vi "FindPlanehs.vi"() -> ()   [LabVIEW 2022 SP3]
uses:
  <vilib>/Utility/file.llb/Write To Spreadsheet File (DBL).vi
  <vilib>/Platform/NI_3dgraph.lvlib
panel:
  in  "Save?":bool
  out "case number":i32[](graph)
  out "outer index":dbl[](array[numeric]) format="%.2f"
  in  "3D Surface":refnum<k7>(container)
  in  "Z Span (+- value range)":cluster{"x":dbl, "span":dbl, "z":dbl}={"x"=4.0, "span"=4.0, "z"=4.0} {"x" format="%.2f"; "z" format="%.2f"; "span" format="%.2f"}
  in  "Points in span":i32=10
  in  "Variables":T1={"sound spd (cm/s)"=150000, "time step (s)"=1e-08} {"time step (s)" format="%.2e"}
  in  "strip":T2={"Radius cm"=9.0, "h (cm)"=2.0, "a (cm)"=4.0} {"Radius cm" format="%.2f"; "a (cm)" format="%.2f"; "h (cm)" format="%.2f"}
  in  "P":cluster{"x cm":dbl, "y cm":dbl, "z cm":dbl}={"x cm"=0.20000000000000018, "y cm"=-4.0, "z cm"=1.4} {"x cm" format="%.2f"; "z cm" format="%.2f"; "y cm" format="%.2f"}
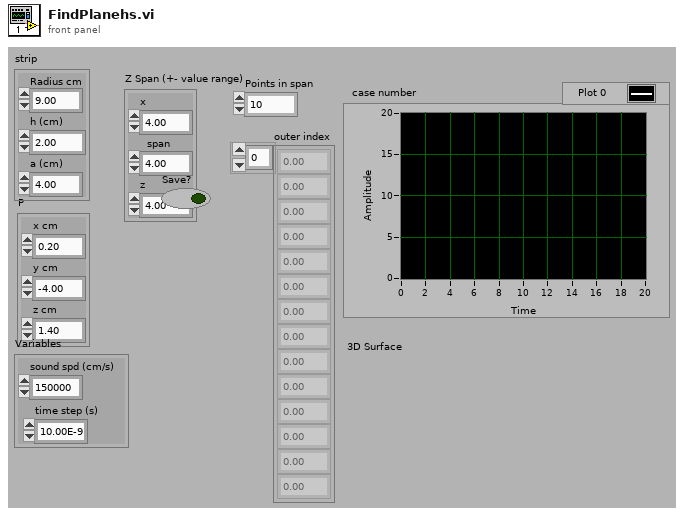
[diagram p1: front panel]
types:
  T1 = cluster{"sound spd (cm/s)":i32, "time step (s)":sgl}
  T2 = cluster{"Radius cm":dbl, "h (cm)":dbl, "a (cm)":dbl}
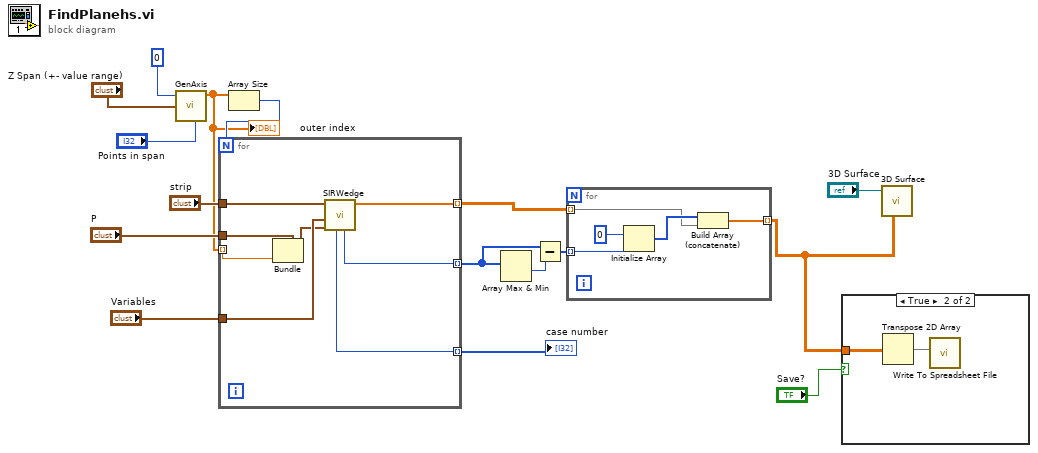
[diagram p0: block diagram]
diagram:
  n1 = call "GenAxis.vi"("Points2"="Points in span", "Plane"=0, "Plane dimensions (cm)"="Z Span (+- value range)") -> ("outer index"=w3:dbl[])  [unwired: 1 in, 3 out]
  "outer index" <- w3
  n2 = Array Size(array=w3) -> (size(s)=w13:i32)
  n3 = for {
    N: w13 -> [_]
    tunnel: "strip" -> [w24]
    tunnel: "Variables" -> [w23]
    tunnel: "P" -> [w22]
    tunnel: w3 -> [w21] mode=indexing
    tunnel: [w19] -> w11 mode=indexing
    tunnel: [w18] -> w10 mode=indexing
    tunnel: [w17] -> w6 mode=indexing
    n4 = Bundle(cluster=w22, "z cm"=w21) -> (w20:cluster{"x cm":dbl, "y cm":dbl, "z cm":dbl})  [unwired: 2 out]
    n5 = call "SIRWedge.vi"("P"=w20, "Variables"=w23, "strip"=w24) -> ("h wedge"=w19:dbl[], "wedge delay"=w18:i32, "Case Number"=w17:i32)  [unwired: 6 out]
  }
  "case number" <- w6
  n6 = Array Max & Min(array=w10) -> (min value=w9:i32)  [unwired: 3 out]
  n7 = Subtract(x=w10, y=w9) -> (x-y=w8:i32[])
  n8 = for {
    tunnel: w11 -> [w26] mode=indexing
    tunnel: w8 -> [w28] mode=indexing
    tunnel: [w25] -> w2 mode=indexing
    n9 = Initialize Array(0, w28) -> (w27:i32[])
    n10 = Build Array (concatenate)(w27, w26) -> (w25:dbl[])
  }
  n11 = case shown="True" "Save?" {
    tunnel: w2 -> [_ w31]
    frame False {
    }
    frame True {
      n12 = Transpose 2D Array(2D array=w31) -> (transposed array=w30:dbl[][])
      n13 = call-poly <vilib>:"Write To Spreadsheet File.vi"("2D data"=w30) -> ()  [unwired: 5 in, 3 out]
    }
  }
  n14 = call <vilib>:"3D Surface.vi"("z matrix"=w2, "3D graph"="3D Surface") -> ()  [unwired: 1 in, 9 out]
